vi "GetPPMSItem.vi"(4 "Fast":bool=TRUE, 5 "Channel":i32=1, 6 "error in (no error)":errorcluster, 7 "Instrument Ref In":refnum<k24>) -> (0 "Result":dbl, 1 "GetPPMSItem Error":i32, 2 "error out":errorcluster, 3 "Instrument Ref Out":refnum<k24>)   [LabVIEW 2016]
uses:
  C:/user/patrick/hg/levylab_inst_ppms2/lvsrc/PPMS2/QDInstrument_LabView/QDInstrument.dll
  QDInstrument.dll
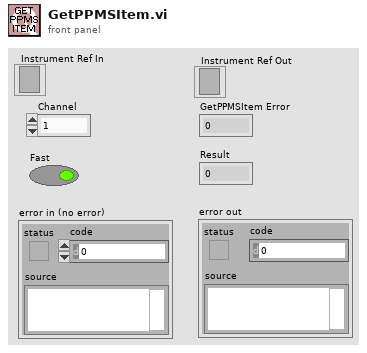
[diagram p1: front panel]
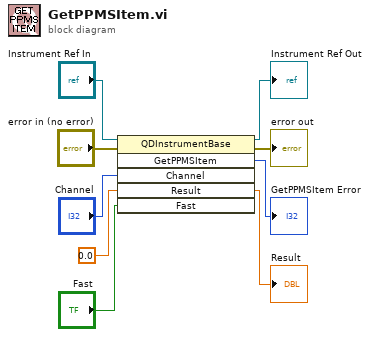
[diagram p0: block diagram]
diagram:
  n1 = invoke class="QDInstrumentBase" method="GetPPMSItem"(reference="Instrument Ref In", error in="error in (no error)", "Channel"="Channel", "Result"=0.0, "Fast"="Fast") -> (reference out=→"Instrument Ref Out":refnum<k24>, error out=→"error out":errorcluster, "GetPPMSItem"=→"GetPPMSItem Error":i32, "Result"=→"Result":dbl)  [unwired: 1 in, 2 out]
